vi "getObstructions.vi"(8 "error in (no error)":errorcluster, 11 "OccupancyMap in":refnum<class "OccupancyMap.lvclass">) -> (0 "error out":errorcluster, 2 "Obstructions":refnum<class "Obstruction.lvclass">[](array[class]), 3 "OccupancyMap out":refnum<class "OccupancyMap.lvclass">)   [LabVIEW 2013, in "OccupancyMap.lvclass"]
uses:
  OccupancyMap.lvclass
  Obstruction/Obstruction.lvclass
  OccupancyMap.lvclass/OccupancyMap.ctl
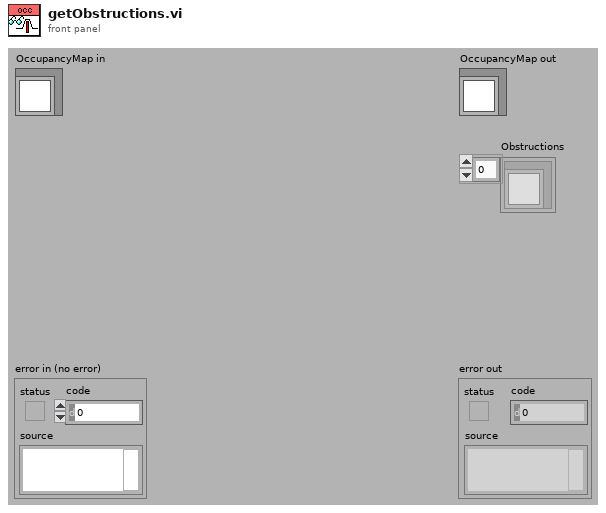
[diagram p1: front panel]
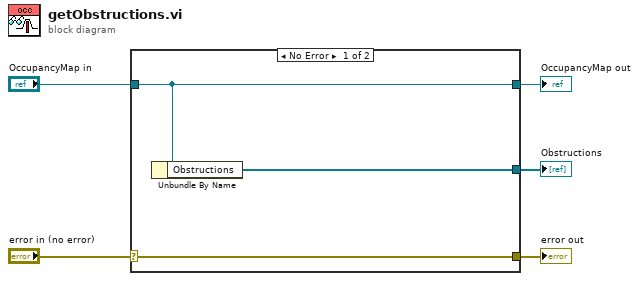
[diagram p0: block diagram]
diagram:
  n1 = case shown="No Error" "error in (no error)" {
    selector: "error in (no error)" -> [w8 w9]
    tunnel: [w8 w9] -> w4
    tunnel: [w7 w10] -> w2
    tunnel: "OccupancyMap in" -> [w7 w10]
    tunnel: [w6 _] -> w1
    frame No Error {
      n2 = Unbundle By Name(w7) -> ("Obstructions"=w6:refnum<class "Obstruction.lvclass">[])
    }
    frame Error {
    }
  }
  "error out" <- w4
  "OccupancyMap out" <- w2
  "Obstructions" <- w1
